vi "Config Dispatcher.vi"(8 "error in (no error)":errorcluster, 10 "Selection":i32, 11 "DataGrid Config Dialog in":refnum<class "DataGrid Config Dialog.lvclass">) -> (0 "error out":errorcluster, 3 "DataGrid Config Dialog out":refnum<class "DataGrid Config Dialog.lvclass">)   [LabVIEW 2018, in "DataGrid Config Dialog.lvclass"]
uses:
  DataGrid Config Dialog.lvclass
  DataGrid Config Dialog.lvclass/DataGrid Config Dialog.ctl
  Data Type Classes/Generic/Generic Data Type.lvclass
  DataGrid Config/DataGrid Config.lvclass
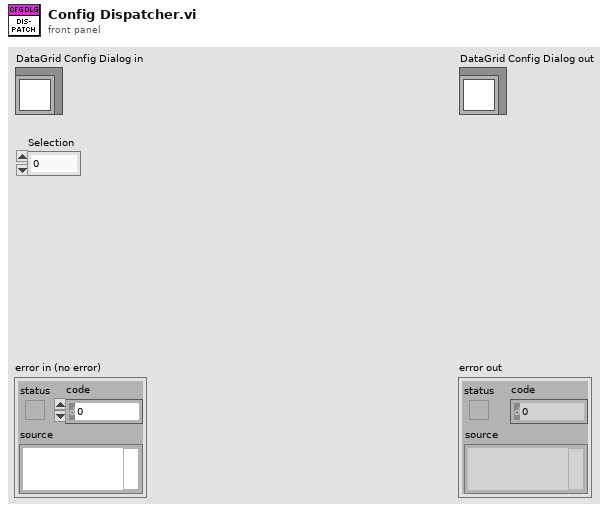
[diagram p1: front panel]
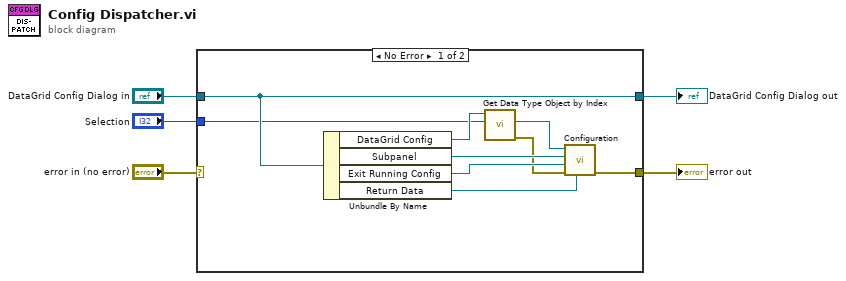
[diagram p0: block diagram]
diagram:
  n1 = case shown="No Error" "error in (no error)" {
    selector: "error in (no error)" -> [_ w16]
    tunnel: [w10 w16] -> w4
    tunnel: [w14 w15] -> w2
    tunnel: "DataGrid Config Dialog in" -> [w14 w15]
    tunnel: "Selection" -> [w8 _]
    frame No Error {
      n2 = Unbundle By Name(w14) -> ("DataGrid Config"=w9:refnum<class "DataGrid Config.lvclass">, "Subpanel"=w13:refnum<class "Panel.lvclass">, "Exit Running Config"=w12:refnum<user-event>, "Return Data"=w11:refnum<user-event>)
      n3 = call "Get Data Type Object by Index.vi"("Index"=w8, "DataGrid Config in"=w9) -> ("error out"=w6:errorcluster, "Data Type Object"=w7:refnum<class "Generic Data Type.lvclass">)  [unwired: 7 in, 1 out]
      n4 = call-dynamic "Configuration.vi"("Return Data"=w11, "error in (no error)"=w6, "Exit Running Config"=w12, "Panel in"=w13, "Generic Data Type in"=w7) -> ("error out"=w10:errorcluster)  [unwired: 5 in, 1 out]
    }
    frame Error {
    }
  }
  "error out" <- w4
  "DataGrid Config Dialog out" <- w2
